vi "Increment Limits Page.vi"(8 "error in (no error)":errorcluster) -> (0 "error out":errorcluster)   [LabVIEW 2009]
uses:
  lib/Data Access Objects/Metadata/Actuator Point.ctl
  lib/Data Access Objects/Metadata/LBCB Number.ctl
  lib/Data Access Objects/Metadata/Cartesian Point.ctl
  Popups/Update Actions.ctl
  lib/Control Loop/Parameters Changes.ctl
  lib/Control Loop/Parameter Change States.ctl
  lib/Data Access Objects/Metadata/Persistant DAO Actions.ctl
  lib/Data Access Objects/Metadata/DAO Actions.ctl
  lib/Launcher/NoPanelAppTypes.ctl
  lib/Launcher/Launcher Actions.ctl
panel:
  in  "Ok":bool
  in  "LBCB Number":T1
  in  "Tab Control":enum32{"Cartesian", "Actuator"}(tab)
  out "Cart Current Incr":dbl[](array[numeric])=[-0.014471871278962644, -0.0027477897622864888, 0.03594582291831433, -0.006177356244415369, -0.000527948512754489, 0.04718526152757189] caption="Current Increments"
  in  "Cart Incr Limit":T2 caption="Increment Limits"
  out "Act Current Incr":dbl[](array[numeric])=[-0.014471871278962644, -0.0027477897622864888, 0.03594582291831433, -0.006177356244415369, -0.000527948512754489, 0.04718526152757189] caption="Current Increments"
  in  "Act Incr Limit":T3 caption="Increment Limits"
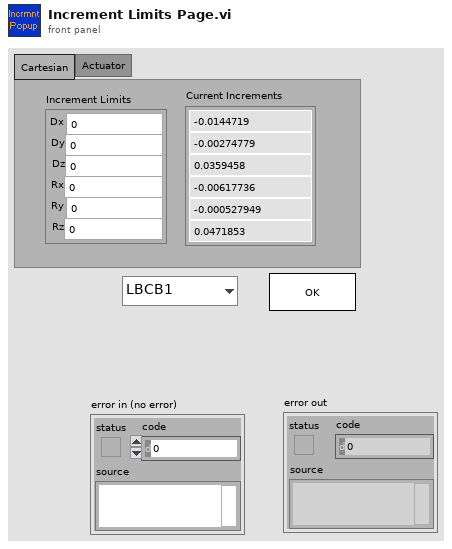
[diagram p1: front panel]
types:
  T1 = typedef "LBCB Number.ctl" = enum16{"LBCB1", "LBCB2"}
  T2 = typedef "Cartesian Point.ctl" = cluster{"Dx":dbl, "Dy":dbl, "Dz":dbl, "Rx":dbl, "Ry":dbl, "Rz":dbl}
  T3 = typedef "Actuator Point.ctl" = cluster{"X1":dbl, "X2":dbl, "Y1":dbl, "Z1":dbl, "Z2":dbl, "Z3":dbl}
  T4 = typedef "Parameters Changes.ctl" = cluster{"Change State":T5, "LBCB Number":T1}
  T5 = typedef "Parameter Change States.ctl" = enum16{"Mixed Mode", "Control Loop", "Limits", "Application", "Stiffness Jacobian", "Start DAQ", "Reset Auto-Balance", "Set Command", "Enable Control", "Disable Control", "Position", "Stop Application"}
  T6 = typedef "Update Actions.ctl" = enum16{"Update", "Exit"}
  T7 = typedef "Persistant DAO Actions.ctl" = enum16{"Init", "Get", "Set", "Load", "Save"}
  T8 = typedef "DAO Actions.ctl" = enum16{"Init", "Get", "Set"}
  T9 = typedef "Act & Cart Commands.ctl" = cluster{"Act Cmd":dbl[], "Cart Cmd":dbl[]}
  T10 = typedef "NoPanelAppTypes.ctl" = enum16{"NTCP Socket", "Data Archiving", "DAQ Link", "Control Loops", "Cmd Disp Diffs", "Individual Readings", "Limits", "Increment Limits"}
  T11 = typedef "Launcher Actions.ctl" = enum16{"Launch", "Stop All", "Stop", "Kill", "Running?", "Init"}
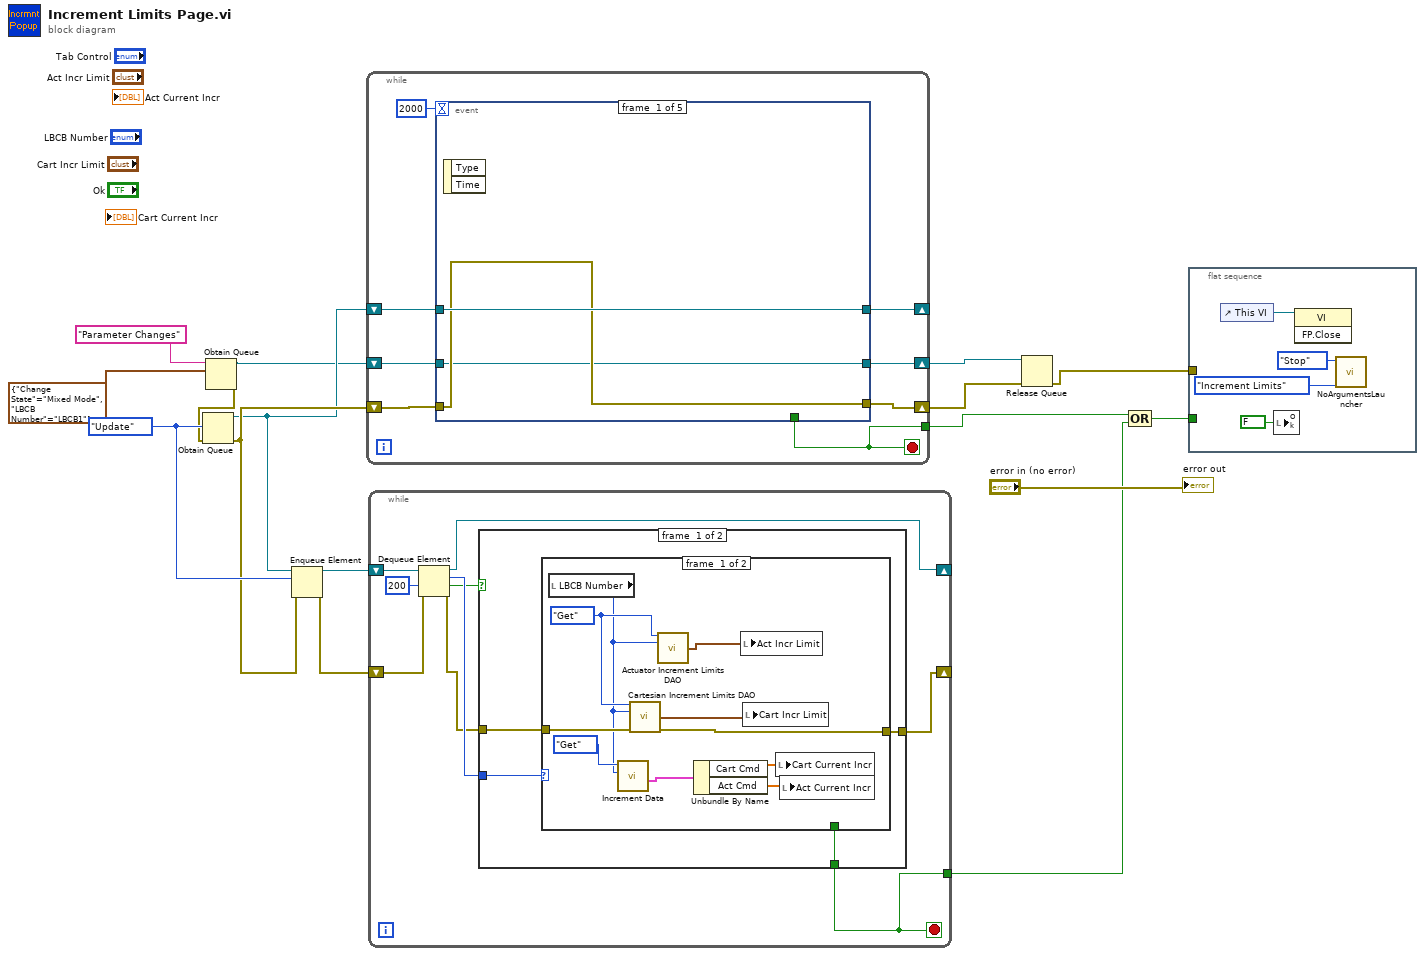
[diagram p0: block diagram]
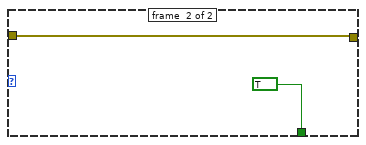
[diagram p2: hidden frame]
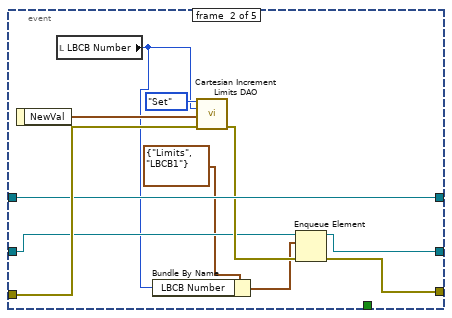
[diagram p4: hidden frame]
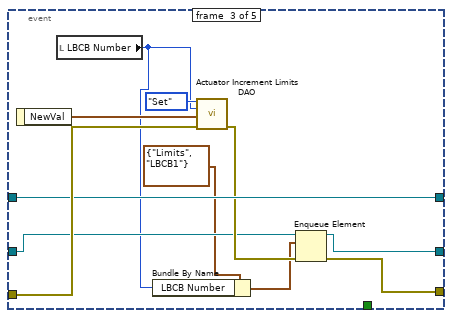
[diagram p5: hidden frame]
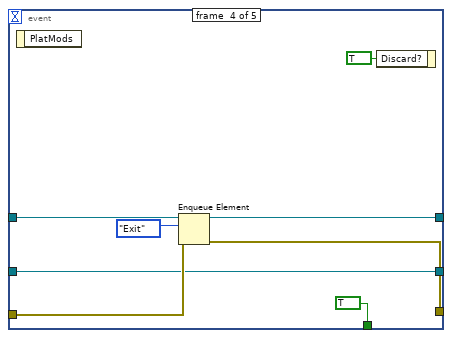
[diagram p6: hidden frame]
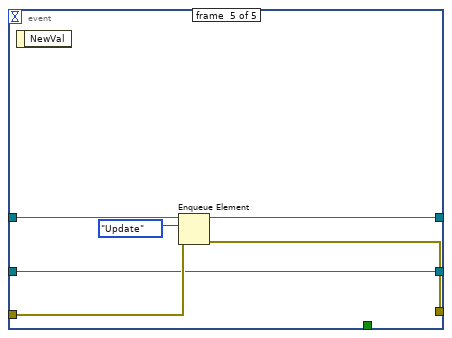
[diagram p7: hidden frame]
diagram:
  w14 = Update_Actions."Update" ("Update Actions")
  n1 = Obtain Queue(name (unnamed)="Parameter Changes", element data type=T4 {"Change State"=enum."Mixed Mode", "LBCB Number"=enum."LBCB1"} ("Parameter Changes")) -> (queue out=w7:refnum<queue>, error out=w8:errorcluster)  [unwired: 3 in, 1 out]
  n2 = Obtain Queue(element data type=w14, error in (no error)=w8) -> (queue out=w12:refnum<queue>, error out=w13:errorcluster)  [unwired: 3 in, 1 out]
  n3 = Enqueue Element(queue=w12, element=w14, error in (no error)=w13) -> (queue out=w16:refnum<queue>, error out=w15:errorcluster)  [unwired: 1 in, 1 out]
  n4 = while {
    shift-right: [w22] -> w5
    shift-left: w13 -> [w23]
    shift-right: [w20] -> _
    shift-left: w12 -> [w21]
    shift-right: [w18] -> w6
    shift-left: w7 -> [w19]
    tunnel: [w17] -> w4
    stop <- w17 stop-if-true
    n5 = event shown="[4] \"LBCB Number\": Value Change" {
      selector: _ -> [_ _ _ _ _]
      dyn-events: _ -> [_ _ _ _ _]
      timeout: 2000 -> [_ _ _ _ _]
      tunnel: w23 -> [w26 w36 w47 w57 w63]
      tunnel: [w26 w28 w39 w56 w62] -> w22
      tunnel: w21 -> [w27 w35 w46 w55 w61]
      tunnel: [w27 w35 w46 w53 w60] -> w20
      tunnel: [_ _ _ TRUE _] -> w17
      tunnel: w19 -> [w25 w33 w44 w50 w58]
      tunnel: [w25 w29 w40 w50 w58] -> w18
      event #0 {
        n6 = event-data() -> ()  [unwired: 1 in, 2 out]
      }
      event #1 {
        n7 = event-data() -> ("NewVal"=w38:T2)  [unwired: 1 in]
        n8 = local read "LBCB Number"() -> (w30:T1)
        n9 = Bundle By Name(cluster=T4 {"Change State"=enum."Limits", "LBCB Number"=enum."LBCB1"} ("element"), "LBCB Number"=w30) -> (w31:T4)
        n10 = call "Cartesian Increment Limits DAO.vi"("Actions"=Persistant_DAO_Actions."Set", "LBCB Number"=w30, "Inc Limits In"=w38, "error in (no error)"=w36) -> ("error out"=w34:errorcluster)  [unwired: 9 in, 2 out]
        n11 = Enqueue Element(queue=w33, element=w31, error in (no error)=w34) -> (queue out=w29:refnum<queue>, error out=w28:errorcluster)  [unwired: 1 in, 1 out]
      }
      event #2 {
        n12 = event-data() -> ("NewVal"=w49:T3)  [unwired: 1 in]
        n13 = local read "LBCB Number"() -> (w41:T1)
        n14 = Bundle By Name(cluster=T4 {"Change State"=enum."Limits", "LBCB Number"=enum."LBCB1"} ("element"), "LBCB Number"=w41) -> (w42:T4)
        n15 = call "Actuator Increment Limits DAO.vi"("Actions"=Persistant_DAO_Actions."Set", "LBCB Number"=w41, "Inc Limits In"=w49, "error in (no error)"=w47) -> ("error out"=w45:errorcluster)  [unwired: 9 in, 2 out]
        n16 = Enqueue Element(queue=w44, element=w42, error in (no error)=w45) -> (queue out=w40:refnum<queue>, error out=w39:errorcluster)  [unwired: 1 in, 1 out]
      }
      event #3 {
        n17 = event-data() -> ()  [unwired: 1 in, 1 out]
        n18 = Enqueue Element(queue=w55, element=Update_Actions."Exit", error in (no error)=w57) -> (queue out=w53:refnum<queue>, error out=w56:errorcluster)  [unwired: 1 in, 1 out]
        n19 = event-data("Discard?"=TRUE) -> ()  [unwired: 1 in, 1 out]
      }
      event #4 {
        n20 = event-data() -> ()  [unwired: 1 in, 1 out]
        n21 = Enqueue Element(queue=w61, element=Update_Actions."Update", error in (no error)=w63) -> (queue out=w60:refnum<queue>, error out=w62:errorcluster)  [unwired: 1 in, 1 out]
      }
    }
  }
  n22 = while {
    shift-right: [w69] -> _
    shift-left: w16 -> [w72]
    shift-right: [w66] -> _
    shift-left: w15 -> [w71]
    tunnel: [w64] -> w3
    stop <- w64 stop-if-true
    n23 = Dequeue Element(queue=w72, timeout in ms (-1)=200, error in (no error)=w71) -> (queue out=w69:refnum<queue>, element=w68:T6, timed out?=w65:bool, error out=w67:errorcluster)
    n24 = case shown="False" w65 {
      tunnel: w68 -> [w76 _]
      tunnel: w67 -> [w75 w89]
      tunnel: [w74 w89] -> w66
      tunnel: [w73 _] -> w64
      frame #0 {
        n25 = case shown="\"Update\"" w76 {
          tunnel: w75 -> [w85 w88]
          tunnel: [w84 w88] -> w74
          tunnel: [_ TRUE] -> w73
          frame #0 {
            w79 = Persistant_DAO_Actions."Get" ("Actions")
            n26 = local read "LBCB Number"() -> (w77:T1)
            n27 = call "Increment Data.vi"("LBCB Number"=w77, "DAO Actions"=DAO_Actions."Get") -> ("Increments Out"=w82:T9)  [unwired: 8 in, 1 out]
            n28 = call "Cartesian Increment Limits DAO.vi"("Actions"=w79, "LBCB Number"=w77, "error in (no error)"=w85) -> ("Inc Limits Out"=w86:T2, "error out"=w84:errorcluster)  [unwired: 10 in, 1 out]
            n29 = call "Actuator Increment Limits DAO.vi"("Actions"=w79, "LBCB Number"=w77) -> ("Inc Limits Out"=w78:T3)  [unwired: 11 in, 2 out]
            n30 = Unbundle By Name(w82) -> ("Cart Cmd"=w81:dbl[], "Act Cmd"=w80:dbl[])
            n31 = local write "Act Incr Limit"(w78) -> ()
            n32 = local write "Cart Incr Limit"(w86) -> ()
            n33 = local write "Cart Current Incr"(w81) -> ()
            n34 = local write "Act Current Incr"(w80) -> ()
          }
          frame #1 {
          }
        }
      }
      frame #1 {
      }
    }
  }
  n35 = Release Queue(queue=w6, error in (no error)=w5) -> (error out=w1:errorcluster)  [unwired: 1 in, 2 out]
  n36 = Compound Arithmetic op=OR(w4, w3) -> (w2:bool)
  n37 = flat-sequence {
    tunnel: w2 -> [_]
    tunnel: w1 -> [_]
    frame #0 {
      n38 = control-ref of="This VI"() -> (w92:refnum<vi>)
      n39 = local write "Ok"(FALSE ("Ok")) -> ()
      n40 = invoke class="VI" method="FP.Close"(reference=w92) -> ()  [unwired: 2 in, 3 out]
      n41 = call "NoArgumentsLauncher.vi"("Application"=NoPanelAppTypes."Increment Limits", "Application Launcher Actions"=Launcher_Actions."Stop") -> ()  [unwired: 8 in, 2 out]
    }
  }
  "error out" <- "error in (no error)"
